vi "Vin_Vout_3C.vi"(6 "Canale uscita":tag="Dev1/ao0", 7 "Fondo Scala AI2 (65)":dbl(ring)=10.0 items=["10"=10.0, "5"=5.0, "0.5"=0.5, "0.05"=0.05], 8 "Fondo Scala AI1 (33)":dbl(ring)=0.05 items=["10"=10.0, "5"=5.0, "0.5"=0.5, "0.05"=0.05], 9 "Fondo Scala AI0 (68)":dbl(ring)=0.5 items=["10"=10.0, "5"=5.0, "0.5"=0.5, "0.05"=0.05], 10 "V in volt":dbl=0.47000000000000003 format="%.5f") -> (0 "V2 medio":dbl=0.020410802672043954 format="%.5f", 1 "sd 1":dbl=6.579572812884434e-05 format="%.5f", 2 "V1 medio":dbl=0.2160543789193946 format="%.5f", 3 "sd 0":dbl=0.0005302170499127453 format="%.5f", 4 "V0 medio":dbl=0.4507249177887913 format="%.5f", 5 "sd 2":dbl=0.0003224996141319774 format="%.5f")   [LabVIEW 2018]
doc: "VIN_VOUT_3C\nlegge 3 canali\nADL 11/2019"
uses:
  <vilib>/DAQmx/write.llb/DAQmx Write (Analog DBL 1Chan 1Samp).vi
  <vilib>/DAQmx/read.llb/DAQmx Read (Analog 1D DBL 1Chan NSamp).vi
  <vilib>/DAQmx/create/channels.llb/DAQmx Create Channel (AO-Voltage-Basic).vi
  <vilib>/DAQmx/configure/timing.llb/DAQmx Timing (Sample Clock).vi
  <vilib>/DAQmx/miscellaneous.llb/DAQmx Fill In Error Info.vi
  <vilib>/DAQmx/create/channels.llb/DAQmx Create Channel (AI-Voltage-Basic).vi
  <vilib>/Analysis/NI_AALBase.lvlib
panel:
  out "Waveform Graph":dbl[][](graph)
  # "RSE: 68, 33, 65"
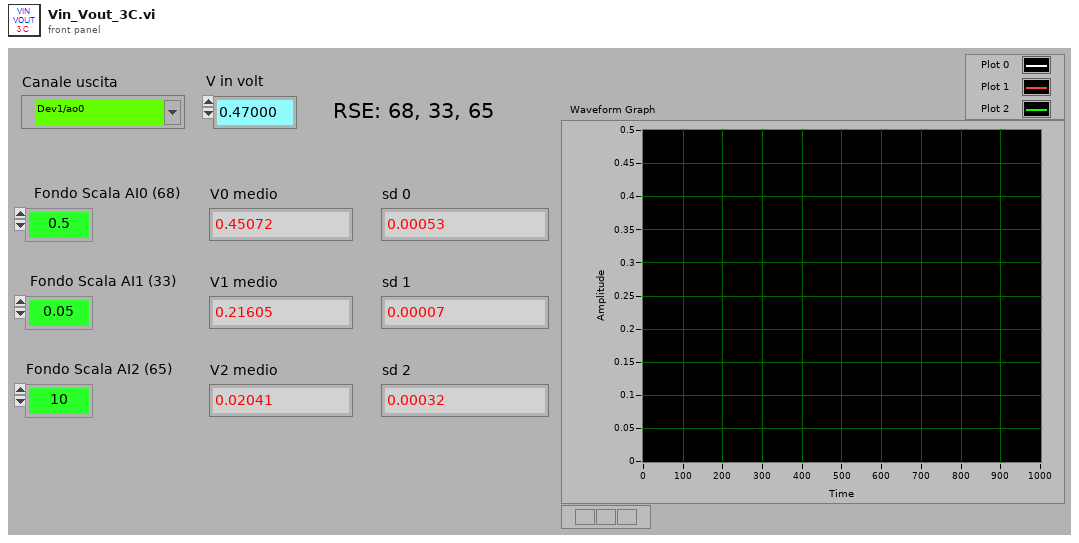
[diagram p1: front panel]
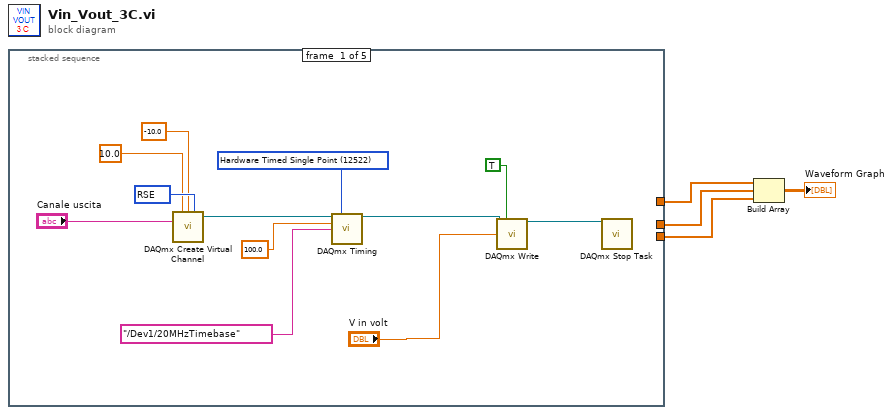
[diagram p0: block diagram]
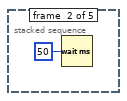
[diagram p2: hidden frame]
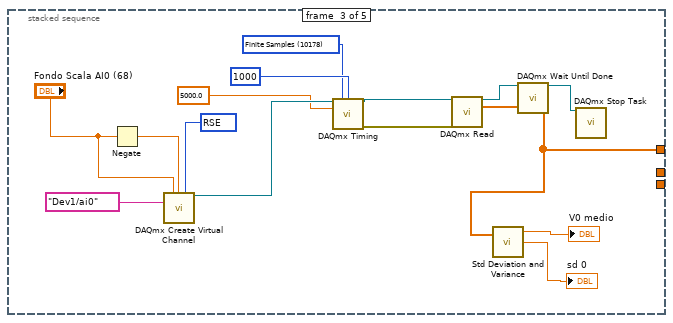
[diagram p3: hidden frame]
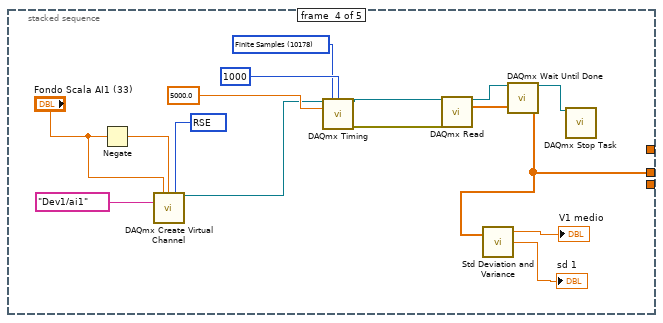
[diagram p4: hidden frame]
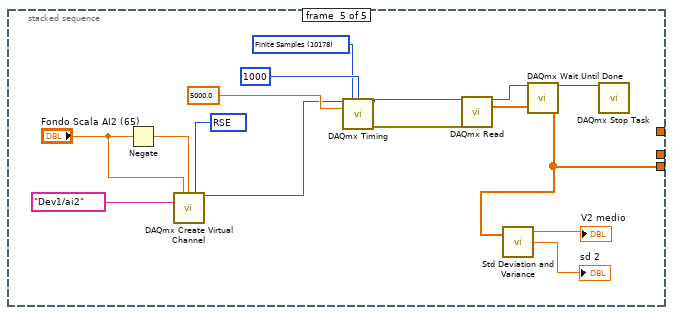
[diagram p5: hidden frame]
diagram:
  n1 = stacked-sequence {
    tunnel: [_ _ w18 _ _] -> w4
    tunnel: [_ _ _ w33 _] -> w3
    tunnel: [_ _ _ _ w48] -> w2
    frame #0 {
      w12 = 12522 items=["Finite Samples"=10178, "Continuous Samples"=10123, "Hardware Timed Single Point"=12522] ("sample mode")
      w16 = 10083 items=["Default"=-1, "RSE"=10083, "Differential"=10106, "Pseudodifferential"=12529] ("output terminal configuration")
      n2 = call-poly <vilib>:"DAQmx Create Virtual Channel.vi"("maximum value"=10.0, "minimum value"=-10.0, "output terminal configuration"=w16, "physical channels"="Canale uscita") -> ("task out"=w8:refnum<k21>)  [unwired: 5 in, 6 out]
      n3 = call-poly <vilib>:"DAQmx Timing.vi"("task/channels in"=w8, "sample mode"=w12, "rate"=100.0, "source"=tag "/Dev1/20MHzTimebase") -> ("task out"=w10:refnum<k21>)  [unwired: 3 in, 8 out]
      n4 = call-poly <vilib>:"DAQmx Write.vi"("task/channels in"=w10, "auto start"=TRUE, "data"="V in volt") -> ("task out"=w9:refnum<k21>)  [unwired: 1 in, 11 out]
      n5 = call <vilib>:"DAQmx Stop Task.vi"("task/channels in"=w9) -> ()  [unwired: 1 in, 14 out]
    }
    frame #1 {
      n6 = Wait (ms)(milliseconds to wait=u32 50) -> ()  [unwired: 1 out]
    }
    frame #2 {
      w23 = 10178 items=["Finite Samples"=10178, "Continuous Samples"=10123, "Hardware Timed Single Point"=12522] ("sample mode")
      w31 = 10083 items=["default"=-1, "RSE"=10083, "NRSE"=10078, "Differential"=10106, "Pseudodifferential"=12529] ("input terminal configuration")
      n7 = Negate(x="Fondo Scala AI0 (68)") -> (-x=w32:dbl)
      n8 = call-poly <vilib>:"DAQmx Create Virtual Channel.vi"("maximum value"="Fondo Scala AI0 (68)", "minimum value"=w32, "input terminal configuration"=w31, "physical channels"=tag "Dev1/ai0") -> ("task out"=w26:refnum<k21>)  [unwired: 5 in, 6 out]
      n9 = call-poly <vilib>:"DAQmx Timing.vi"("task/channels in"=w26, "sample mode"=w23, "samples per channel"=u32 1000, "rate"=5000.0) -> ("task out"=w29:refnum<k21>, "error out"=w28:errorcluster)  [unwired: 3 in, 7 out]
      n10 = call-poly <vilib>:"DAQmx Read.vi"("task/channels in"=w29, "error in"=w28) -> ("task out"=w24:refnum<k21>, "data"=w18:dbl[])  [unwired: 1 in, 11 out]
      n11 = call <vilib>:"Std Deviation and Variance.vi"("X"=w18) -> ("mean"=→"V0 medio":dbl, "standard deviation"=→"sd 0":dbl)  [unwired: 1 in, 1 out]
      n12 = call <vilib>:"DAQmx Wait Until Done.vi"("task/channels in"=w24) -> ("task out"=w22:refnum<k21>)  [unwired: 2 in, 12 out]
      n13 = call <vilib>:"DAQmx Stop Task.vi"("task/channels in"=w22) -> ()  [unwired: 1 in, 14 out]
    }
    frame #3 {
      w39 = 10178 items=["Finite Samples"=10178, "Continuous Samples"=10123, "Hardware Timed Single Point"=12522] ("sample mode")
      w46 = 10083 items=["default"=-1, "RSE"=10083, "NRSE"=10078, "Differential"=10106, "Pseudodifferential"=12529] ("input terminal configuration")
      n14 = Negate(x="Fondo Scala AI1 (33)") -> (-x=w47:dbl)
      n15 = call-poly <vilib>:"DAQmx Create Virtual Channel.vi"("maximum value"="Fondo Scala AI1 (33)", "minimum value"=w47, "input terminal configuration"=w46, "physical channels"=tag "Dev1/ai1") -> ("task out"=w34:refnum<k21>)  [unwired: 5 in, 6 out]
      n16 = call-poly <vilib>:"DAQmx Timing.vi"("task/channels in"=w34, "sample mode"=w39, "samples per channel"=u32 1000, "rate"=5000.0) -> ("task out"=w44:refnum<k21>, "error out"=w43:errorcluster)  [unwired: 3 in, 7 out]
      n17 = call-poly <vilib>:"DAQmx Read.vi"("task/channels in"=w44, "error in"=w43) -> ("task out"=w40:refnum<k21>, "data"=w33:dbl[])  [unwired: 1 in, 11 out]
      n18 = call <vilib>:"Std Deviation and Variance.vi"("X"=w33) -> ("mean"=→"V1 medio":dbl, "standard deviation"=→"sd 1":dbl)  [unwired: 1 in, 1 out]
      n19 = call <vilib>:"DAQmx Wait Until Done.vi"("task/channels in"=w40) -> ("task out"=w38:refnum<k21>)  [unwired: 2 in, 12 out]
      n20 = call <vilib>:"DAQmx Stop Task.vi"("task/channels in"=w38) -> ()  [unwired: 1 in, 14 out]
    }
    frame #4 {
      w56 = 10178 items=["Finite Samples"=10178, "Continuous Samples"=10123, "Hardware Timed Single Point"=12522] ("sample mode")
      w62 = 10083 items=["default"=-1, "RSE"=10083, "NRSE"=10078, "Differential"=10106, "Pseudodifferential"=12529] ("input terminal configuration")
      n21 = Negate(x="Fondo Scala AI2 (65)") -> (-x=w51:dbl)
      n22 = call-poly <vilib>:"DAQmx Create Virtual Channel.vi"("maximum value"="Fondo Scala AI2 (65)", "minimum value"=w51, "input terminal configuration"=w62, "physical channels"=tag "Dev1/ai2") -> ("task out"=w55:refnum<k21>)  [unwired: 5 in, 6 out]
      n23 = call-poly <vilib>:"DAQmx Timing.vi"("task/channels in"=w55, "sample mode"=w56, "samples per channel"=u32 1000, "rate"=5000.0) -> ("task out"=w61:refnum<k21>, "error out"=w60:errorcluster)  [unwired: 3 in, 7 out]
      n24 = call-poly <vilib>:"DAQmx Read.vi"("task/channels in"=w61, "error in"=w60) -> ("task out"=w57:refnum<k21>, "data"=w48:dbl[])  [unwired: 1 in, 11 out]
      n25 = call <vilib>:"Std Deviation and Variance.vi"("X"=w48) -> ("mean"=→"V2 medio":dbl, "standard deviation"=→"sd 2":dbl)  [unwired: 1 in, 1 out]
      n26 = call <vilib>:"DAQmx Wait Until Done.vi"("task/channels in"=w57) -> ("task out"=w49:refnum<k21>)  [unwired: 2 in, 12 out]
      n27 = call <vilib>:"DAQmx Stop Task.vi"("task/channels in"=w49) -> ()  [unwired: 1 in, 14 out]
    }
  }
  n28 = Build Array(w4, w3, w2) -> (→"Waveform Graph":dbl[][])
